vi "rqcBob Define Detection Window.vi"(0 "detector.detection cycle length":u8, 5 "detector.detector window in":u8) -> (6 "detector.detector window out":u16)   [LabVIEW 2018]
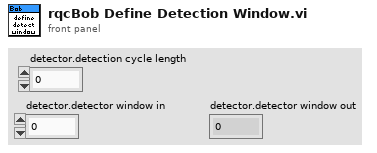
[diagram p1: front panel]
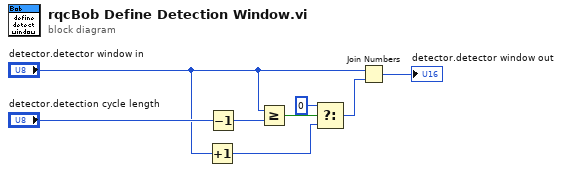
[diagram p0: block diagram]
diagram:
  n1 = Increment(x="detector.detector window in") -> (x+1=w6:u8)
  n2 = Decrement(x="detector.detection cycle length") -> (x-1=w7:u8)
  n3 = Greater Or Equal?(x="detector.detector window in", y=w7) -> (x >= y?=w4:bool)
  n4 = Select(t=u8 0 ("y"), s=w4, f=w6) -> (s? t:f=w2:u8)
  n5 = Join Numbers(hi="detector.detector window in", lo=w2) -> ((hi.lo)=→"detector.detector window out":u16)
